vi "Initialize.vi"(8 "error in (no error)":errorcluster) -> (0 "error out":errorcluster)   [LabVIEW 2025, in "Automotive Ethernet Bus Monitor UI.lvlib" / "lvwpcap.lvlib"]
doc: "This VI initializes the packet sniffer routine."
uses:
  lvwpcap.lvlib
  lvwpcap.dll
panel:
  # "Select Help»Show Context Help and move the cursor over the VI icon to display help for this VI."
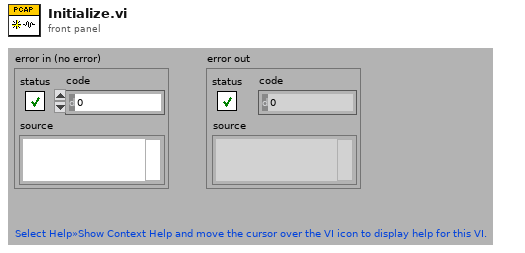
[diagram p1: front panel]
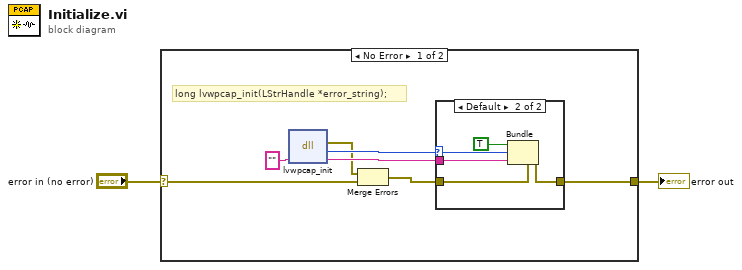
[diagram p0: block diagram]
diagram:
  n1 = case shown="No Error" "error in (no error)" {
    selector: "error in (no error)" -> [w6 w16]
    tunnel: [w7 w16] -> w2
    frame No Error {
      # "long lvwpcap_init(LStrHandle *error_string);"
      n2 = dll-call lib="lvwpcap.*" fn="lvwpcap_init"("error_string"="") -> (error out=w4:errorcluster, "return type"=w9:i32, "error_string"=w8:string)  [unwired: 3 in, 1 out]
      n3 = Merge Errors(w4, w6) -> (w5:errorcluster)
      n4 = case shown="Default" w9 {
        selector: w9 -> [_ w14]
        tunnel: w8 -> [_ w13]
        tunnel: w5 -> [w10 w15]
        tunnel: [w10 w11] -> w7
        frame 0 {
        }
        frame Default {
          n5 = Bundle(cluster=w15, "status"=TRUE, "code"=w14, "source"=w13) -> (w11:errorcluster)
        }
      }
    }
    frame Error {
    }
  }
  "error out" <- w2
